vi "HelpMessage.vi"(11 "ExecuteBuildSpecAllTargets in":refnum<class "ExecuteBuildSpecAllTargets.lvclass">) -> (2 "Help":string, 3 "ExecuteBuildSpecAllTargets out":refnum<class "ExecuteBuildSpecAllTargets.lvclass">)   [LabVIEW 2014, in "ExecuteBuildSpecAllTargets.lvclass"]
uses:
  ExecuteBuildSpecAllTargets.lvclass
panel:
  in  "HelpText":string="LabVIEWCLI -OperationName ExecuteBuildSpecAllTargets -ProjectPath <path of LabVIEW project> -BuildSpecName <name of the build specification>\n\n -ProjectPath : Specifies the full path to the LabVIEW project (.lvproj) file that contains the build specifications.\n -BuildSpecName : Specifies the name of the build specification. Enter the name that appears under Build Specifications in the Project Explorer window to specify which build specification builds. Any build specification in the project matching this name will be built.\n"
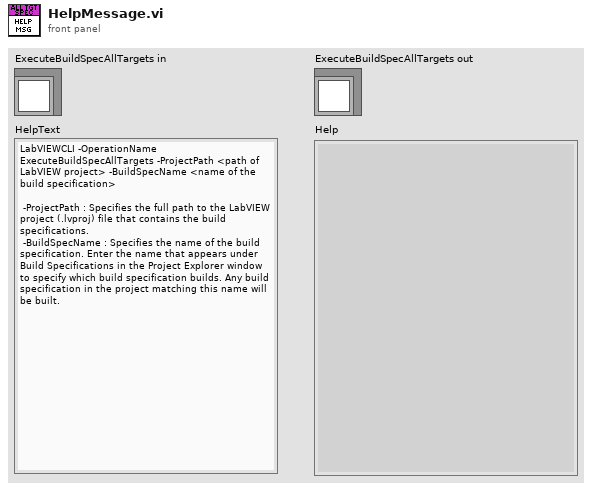
[diagram p1: front panel]
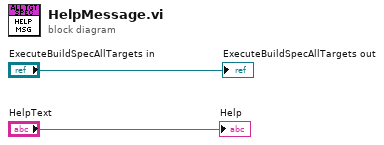
[diagram p0: block diagram]
diagram:
  "ExecuteBuildSpecAllTargets out" <- "ExecuteBuildSpecAllTargets in"
  "Help" <- "HelpText"
